vi "Configure Zone.vi"(0 "VISA resource name":refnum<visa-resource-name>, 1 "Heater Output (1:1)":u16(ring)=1 items=["1"=1, "2"=2], 2 "Zone (1)":dbl=1.0, 3 "Upper Boundary (0.0000)":dbl format="%.3f", 4 "Rate (D) (0 %)":dbl format="%.1f", 5 "error in (no error)":errorcluster, 6 "Gain (P) (50.0)":dbl=50.0 format="%.1f", 7 "Input (0:Default - Previously Assigned)":u16(ring) items=["Default - Previously Assigned", "Input A", "Input B"], 8 "Manual Output (0.000 %)":dbl format="%.2f", 9 "Reset (I) (20.0)":dbl=20.0 format="%.1f", 10 "Heater Range (0:Off)":u16(ring) items=["Off", "Low", "Medium", "High"], 12 "Ramp Rate (0.0 %)":dbl format="%.1f") -> (14 "VISA resource name out":refnum<visa-resource-name>, 19 "error out":errorcluster)   [LabVIEW 2014, in "Lake Shore 335.lvlib"]
doc: "Configures the parameters of a control loop's zone table. The Model 335 allows the user to establish up to 10 custom contiguous temperature zones where the controller will automatically use the pre-programmed PID values and heater ranges. Zone control can be active for both control loops at the same time. To use the programmed zones, the output mode must be set to Zone."
uses:
  Lake Shore 335.lvlib
  Instance           1 22Saved   Configure Zone .vi
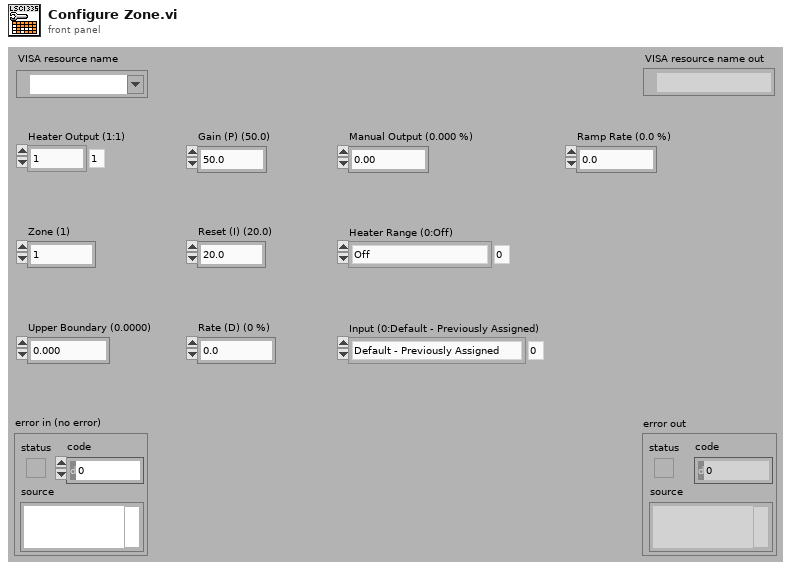
[diagram p1: front panel]
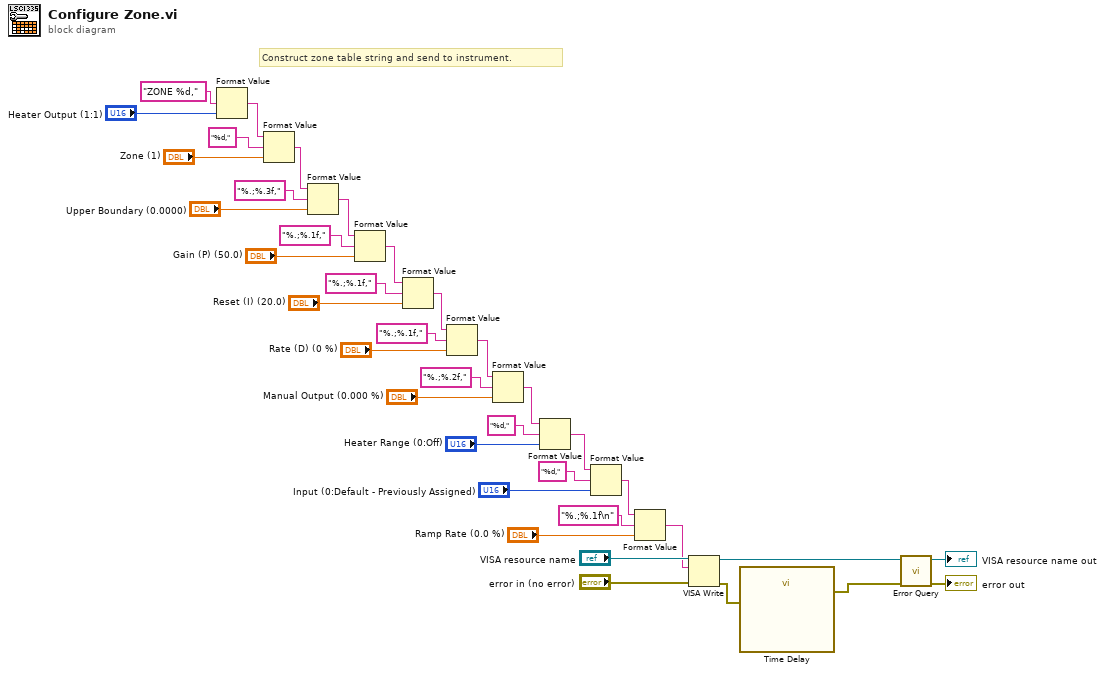
[diagram p0: block diagram]
diagram:
  # "Construct zone table string and send to instrument."
  n1 = Format Value(format string="ZONE %d,", value (0)="Heater Output (1:1)") -> (output string=w21:string)  [unwired: 1 in]
  n2 = Format Value(string ("")=w21, format string="%d,", value (0)="Zone (1)") -> (output string=w23:string)
  n3 = Format Value(string ("")=w23, format string="%.;%.3f,", value (0)="Upper Boundary (0.0000)") -> (output string=w27:string)
  n4 = Format Value(string ("")=w27, format string="%.;%.1f,", value (0)="Gain (P) (50.0)") -> (output string=w28:string)
  n5 = Format Value(string ("")=w28, format string="%.;%.1f,", value (0)="Reset (I) (20.0)") -> (output string=w29:string)
  n6 = Format Value(string ("")=w29, format string="%.;%.1f,", value (0)="Rate (D) (0 %)") -> (output string=w30:string)
  n7 = Format Value(string ("")=w30, format string="%.;%.2f,", value (0)="Manual Output (0.000 %)") -> (output string=w20:string)
  n8 = Format Value(string ("")=w20, format string="%d,", value (0)="Heater Range (0:Off)") -> (output string=w14:string)
  n9 = Format Value(string ("")=w14, format string="%d,", value (0)="Input (0:Default - Previously Assigned)") -> (output string=w12:string)
  n10 = Format Value(string ("")=w12, format string="%.;%.1f\n", value (0)="Ramp Rate (0.0 %)") -> (output string=w11:string)
  n11 = VISA Write(VISA resource name="VISA resource name", write buffer=w11, error in (no error)="error in (no error)") -> (VISA resource name out=w32:refnum<visa-resource-name>, error out=w16:errorcluster)  [unwired: 1 out]
  n12 = call "Time Delay"("error in (no error)"=w16) -> ("error out"=w33:errorcluster)  [unwired: 10 in]
  n13 = call "Error Query.vi"("error in (no error)"=w33, "VISA resource name"=w32) -> ("error out"=→"error out":errorcluster, "VISA resource name out"=→"VISA resource name out":refnum<visa-resource-name>)  [unwired: 7 in, 1 out]
